vi "Language(FGV).vi"(10 "Language in":string, 11 "OP":enum16{"GET", "SET"}(ring)) -> (2 "Language out":string)   [LabVIEW 2019, in "Localization.lvlib"]
uses:
  Localization.lvlib
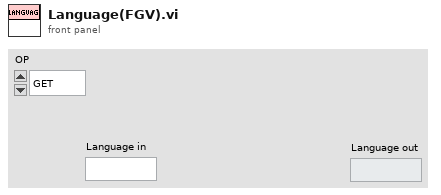
[diagram p1: front panel]
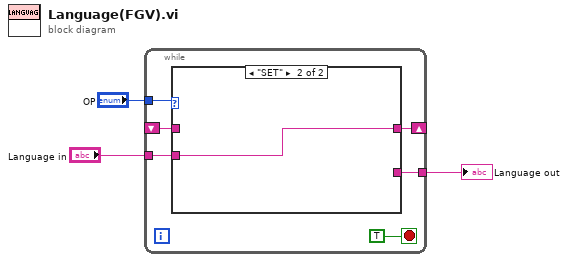
[diagram p0: block diagram]
diagram:
  n1 = while {
    shift-right: [w7] -> _
    shift-left: _ -> [w6]
    tunnel: "OP" -> [w8]
    tunnel: [w5] -> w2
    tunnel: "Language in" -> [w4]
    stop <- TRUE stop-if-true
    n2 = case shown="\"SET\"" w8 {
      tunnel: [w10 w11] -> w7
      tunnel: w6 -> [w10 _]
      tunnel: [w10 _] -> w5
      tunnel: w4 -> [_ w11]
      frame "GET", Default {
      }
      frame "SET" {
      }
    }
  }
  "Language out" <- w2
